vi "Initialize.vi"(8 "error in":errorcluster, 10 "sPanel":refnum<vi>, 11 "cPAS Facade in":refnum<class "cPAS Facade.lvclass">) -> (0 "error out":errorcluster, 3 "cPAS Facade out":refnum<class "cPAS Facade.lvclass">)   [LabVIEW 2012, in "cPAS Facade.lvclass"]
doc: "The initialize function is abstract as the layout will be dependent on the implementation."
uses:
  cPAS Facade.lvclass
  Reusable/GUI/Composition/GUI Composition.lvclass
  Reusable/GUI/GUI.lvclass
  Reusable/Observer/Data Subject.lvclass
  PAS/Class/PAS/Controls/PAS Control.lvclass
  PAS/Class/PAS/HF UI/PAS HF UI.lvclass
  PAS/Class/PAS/Derived/PAS Derived.lvclass
  CRDS/Controls/CRD Controls.lvclass
  CRDS/Ringdowns/CRD Ringdowns.lvclass
  CRDS/Derived Data/CRD Derived.lvclass
  Observer/cPAS Subject.lvclass
  CRDS/Subject/CRD Subject.lvclass
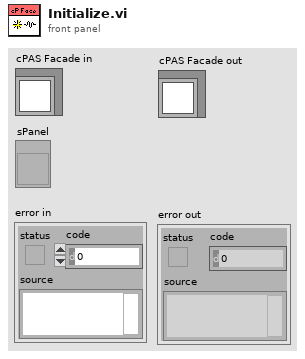
[diagram p1: front panel]
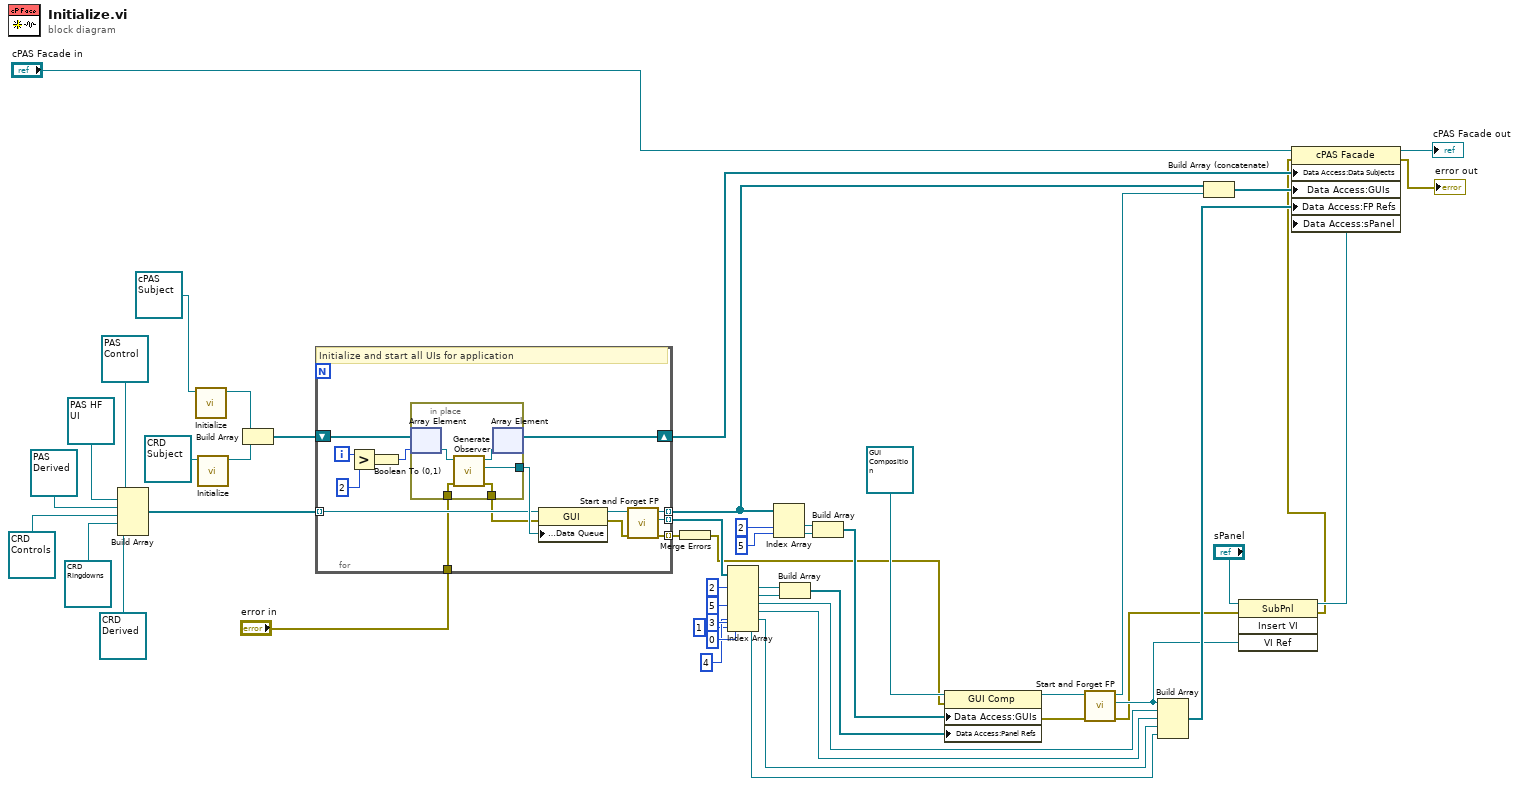
[diagram p0: block diagram]
diagram:
  n1 = Build Array(refnum<class "PAS Control.lvclass"> refnum ("PAS Control"), refnum<class "PAS HF UI.lvclass"> refnum ("PAS HF UI"), refnum<class "PAS Derived.lvclass"> refnum ("PAS Derived.lvclass"), refnum<class "CRD Controls.lvclass"> refnum ("CRD Ctl UI"), refnum<class "CRD Ringdowns.lvclass"> refnum ("CRD Ringdowns.lvclass"), refnum<class "CRD Derived.lvclass"> refnum ("CRD Derived.lvclass")) -> (w47:refnum<class "GUI.lvclass">[])
  n2 = call-dynamic "Initialize.vi"("cPAS Subject in"=refnum<class "cPAS Subject.lvclass"> refnum ("cPAS Subj")) -> ("cPAS Subject out"=w38:refnum<class "cPAS Subject.lvclass">)  [unwired: 8 in, 2 out]
  n3 = call-dynamic "Initialize.vi"("CRD Subject in"=refnum<class "CRD Subject.lvclass"> refnum ("CRD Subj")) -> ("CRD Subject out"=w36:refnum<class "CRD Subject.lvclass">)  [unwired: 8 in, 2 out]
  n4 = Build Array(w38, w36) -> (w40:refnum<class "Data Subject.lvclass">[])
  n5 = for {
    tunnel: w47 -> [w56] mode=indexing
    shift-right: [w57] -> w14
    shift-left: w40 -> [w63]
    tunnel: [w54] -> w35 mode=indexing
    tunnel: [w53] -> w17 mode=indexing
    tunnel: [w52] -> w2 mode=indexing
    tunnel: "error in" -> [w51]
    i -> [w65]
    # "Initialize and start all UIs for application"
    n6 = Greater?(x=w65, y=2) -> (0:w62:bool)
    n7 = Boolean To (0,1)(Boolean=w62) -> (0, 1=w61:i16)
    n8 = in-place {
      in-place-border: [w68] -> w58
      in-place-border: [w67] -> w55
      in-place-border: w51 -> [w66]
      n9 = in-place-array #1(w63, w61) -> (w70:refnum<class "Data Subject.lvclass">)
      n10 = call "Generate Observer.vi"("error in"=w66, "Data Subject in"=w70) -> ("error out"=w67:errorcluster, "Observer"=w68:refnum<queue>, "Data Subject out"=w69:refnum<class "Data Subject.lvclass">)  [unwired: 7 in]
      n11 = in-place-array #1(w69) -> (w57:refnum<class "Data Subject.lvclass">[])  [unwired: 1 out]
    }
    n12 = property class="GUI"(reference=w56, error in=w55, "Data Access:Data Queue"=w58) -> (reference out=w59:refnum<class "GUI.lvclass">, error out=w60:errorcluster)
    n13 = call-dynamic "Start and Forget FP.vi"("error in"=w60, "GUI in"=w59) -> ("error out"=w52:errorcluster, "UI Ref"=w54:refnum<vi>, "GUI out"=w53:refnum<class "GUI.lvclass">)  [unwired: 6 in, 1 out]
  }
  n14 = Merge Errors(w2) -> (w1:errorcluster)
  n15 = Index Array(array=w35, index #1=2 ("index"), index #2=5 ("index"), index #3=3 ("index"), index #4=0 ("index"), index #5=4 ("index"), index #6=1 ("index")) -> (element #1=w28:refnum<vi>, element #2=w27:refnum<vi>, element #3=w23:refnum<vi>, element #4=w22:refnum<vi>, element #5=w18:refnum<vi>, element #6=w11:refnum<vi>)
  n16 = Index Array(array=w17, index #1=2 ("index"), index #2=5 ("index")) -> (element #1=w30:refnum<class "GUI.lvclass">, element #2=w29:refnum<class "GUI.lvclass">)
  n17 = Build Array(w28, w27) -> (w26:refnum<vi>[])
  n18 = Build Array(w30, w29) -> (w25:refnum<class "GUI.lvclass">[])
  n19 = property class="GUI Comp"(reference=refnum<class "GUI Composition.lvclass"> refnum ("GUI Composition.lvclass"), error in=w1, "Data Access:GUIs"=w25, "Data Access:Panel Refs"=w26) -> (reference out=w49:refnum<class "GUI Composition.lvclass">, error out=w48:errorcluster)
  n20 = call-dynamic "Start and Forget FP.vi"("error in"=w48, "GUI in"=w49) -> ("error out"=w5:errorcluster, "UI Ref"=w6:refnum<vi>, "GUI out"=w16:refnum<class "GUI Composition.lvclass">)  [unwired: 6 in, 1 out]
  n21 = Build Array(w6, w23, w22, w18, w11) -> (w12:refnum<vi>[])
  n22 = Build Array (concatenate)(w17, w16) -> (w13:refnum<class "GUI.lvclass">[])
  n23 = invoke class="SubPnl" method="Insert VI"(reference="sPanel", error in=w5, "VI Ref"=w6) -> (reference out=w4:refnum<vi>, error out=w3:errorcluster)  [unwired: 1 in, 2 out]
  n24 = property class="cPAS Facade"(reference="cPAS Facade in", error in=w3, "Data Access:Data Subjects"=w14, "Data Access:GUIs"=w13, "Data Access:FP Refs"=w12, "Data Access:sPanel"=w4) -> (reference out=→"cPAS Facade out":refnum<class "cPAS Facade.lvclass">, error out=→"error out":errorcluster)
